vi "pattern_matching_mit_thresholding.vi"() -> ()   [LabVIEW 2014]
uses:
  <vilib>/vision/driver/NI_Vision_Acquisition_Software.lvlib
  <vilib>/userdefined/High Color/IMAQdx.ctl
  <vilib>/vision/NI_Vision_Development_Module.lvlib
  <vilib>/vision/Avi1.llb/AviRefnum.ctl
  <resource>/objmgr/imaqdx.rc
  subvis/Control 1.ctl
panel:
  in  "Replace Value":sgl=1.0 format="%.2f"
  in  "Keep/Replace Value (Replace)":bool=TRUE
  in  "Range":cluster{"Lower value":sgl, "Upper value":sgl}={"Lower value"=128.0, "Upper value"=255.0} {"Upper value" format="%.2f"; "Lower value" format="%.2f"}
  in  "Länge der Spur":i32=50
  in  "Frames Per Second":u32=20
  in  "BayerPattern":u32(ring)=5 items=["None", "GB", "GR", "BG", "RG", "Use Hardware Value"]
  in  "ValueString 2":T1="BayerGB8"
  out "ValueString":string
  out "ValueBool":bool
  out "IPAddress":string
  in  "y":i32
  in  "x":i32
  in  "Pattern2 Farbe":u32(colorbox)=16711680
  in  "pattern3":bool
  in  "y 3":i32
  in  "x 3":i32
  out "Pattern 5":T2(plugin-control)
  in  "Pattern5 Farbe":u32(colorbox)=16711680
  in  "pattern5":bool
  in  "y 5":i32
  in  "x 5":i32
  in  "Pattern4 Farbe":u32(colorbox)=16711680
  in  "pattern4":bool
  in  "y 4":i32
  in  "x 4":i32
  out "Pattern 4":T2(plugin-control)
  in  "Template File Path (Pattern Matching 4":path=path "C:/Users/Kroll/Desktop/Test_04012016/Pattern/templet_invertiert_2.png"
  in  "Template File Path (Pattern Matching 5":path=path "C:/Users/Kroll/Desktop/Test_04012016/Pattern/TEST_PAINT.png"
  in  "Pattern2 Farbe":u32(colorbox)=16711680
  in  "pattern2":bool
  out "Pattern 3":T2(plugin-control)
  in  "Template File Path (Pattern Matching 3":path=path "C:/Users/Kroll/Desktop/Test_04012016/Pattern/pattern3.png"
  out "Pattern1":T2(plugin-control)
  out "Pattern 2":T2(plugin-control)
  in  "Pattern1 Farbe":u32(colorbox)=16711680
  in  "pattern1":bool
  out "Acquired Frames/s":dbl
  in  "Länge des Pfeils":sgl=80.0
  in  "Aufnahme Starten":bool
  out "Selected Path":path
  in  "Max Data Size":u32=10000
  in  "y 2":i32
  in  "x 2":i32
  out "Processed Frames/s":dbl
  in  "Template File Path (Pattern Matching 2":path=path "C:/Users/Kroll/Desktop/Test_04012016/Pattern/pattern_test_1412.png"
  in  "millisecond multiple":u32
  in  "Mittelpunktgröße":sgl
  out "date/time string":string
  in  "file path (dialog if empty)":path=path "I:/123.txt"
  in  "Template File Path (Pattern Matching 1)":path=path "C:/Users/Kroll/Desktop/Test_04012016/Pattern/pattern_1412.png"
  in  "Parameters Pattern":T3={"Number of Matches Requested"=1, "Minimum Match Score"=800.0, "Angle Ranges"=[{"Start Angle"=-180.0, "End Angle"=180.0}, {"Start Angle"=0.0, "End Angle"=360.0}]}
  in  "Programm anhalten":bool
  out "Threshold Image 2":T2(plugin-control)
  out "Image 2":T2(plugin-control)
  # "Speicherort der Log Datei"
  # "Program Delay einstellen"
  # "Zum Rauszoomen Shift benutzen ->"
  # "Aufnahme"
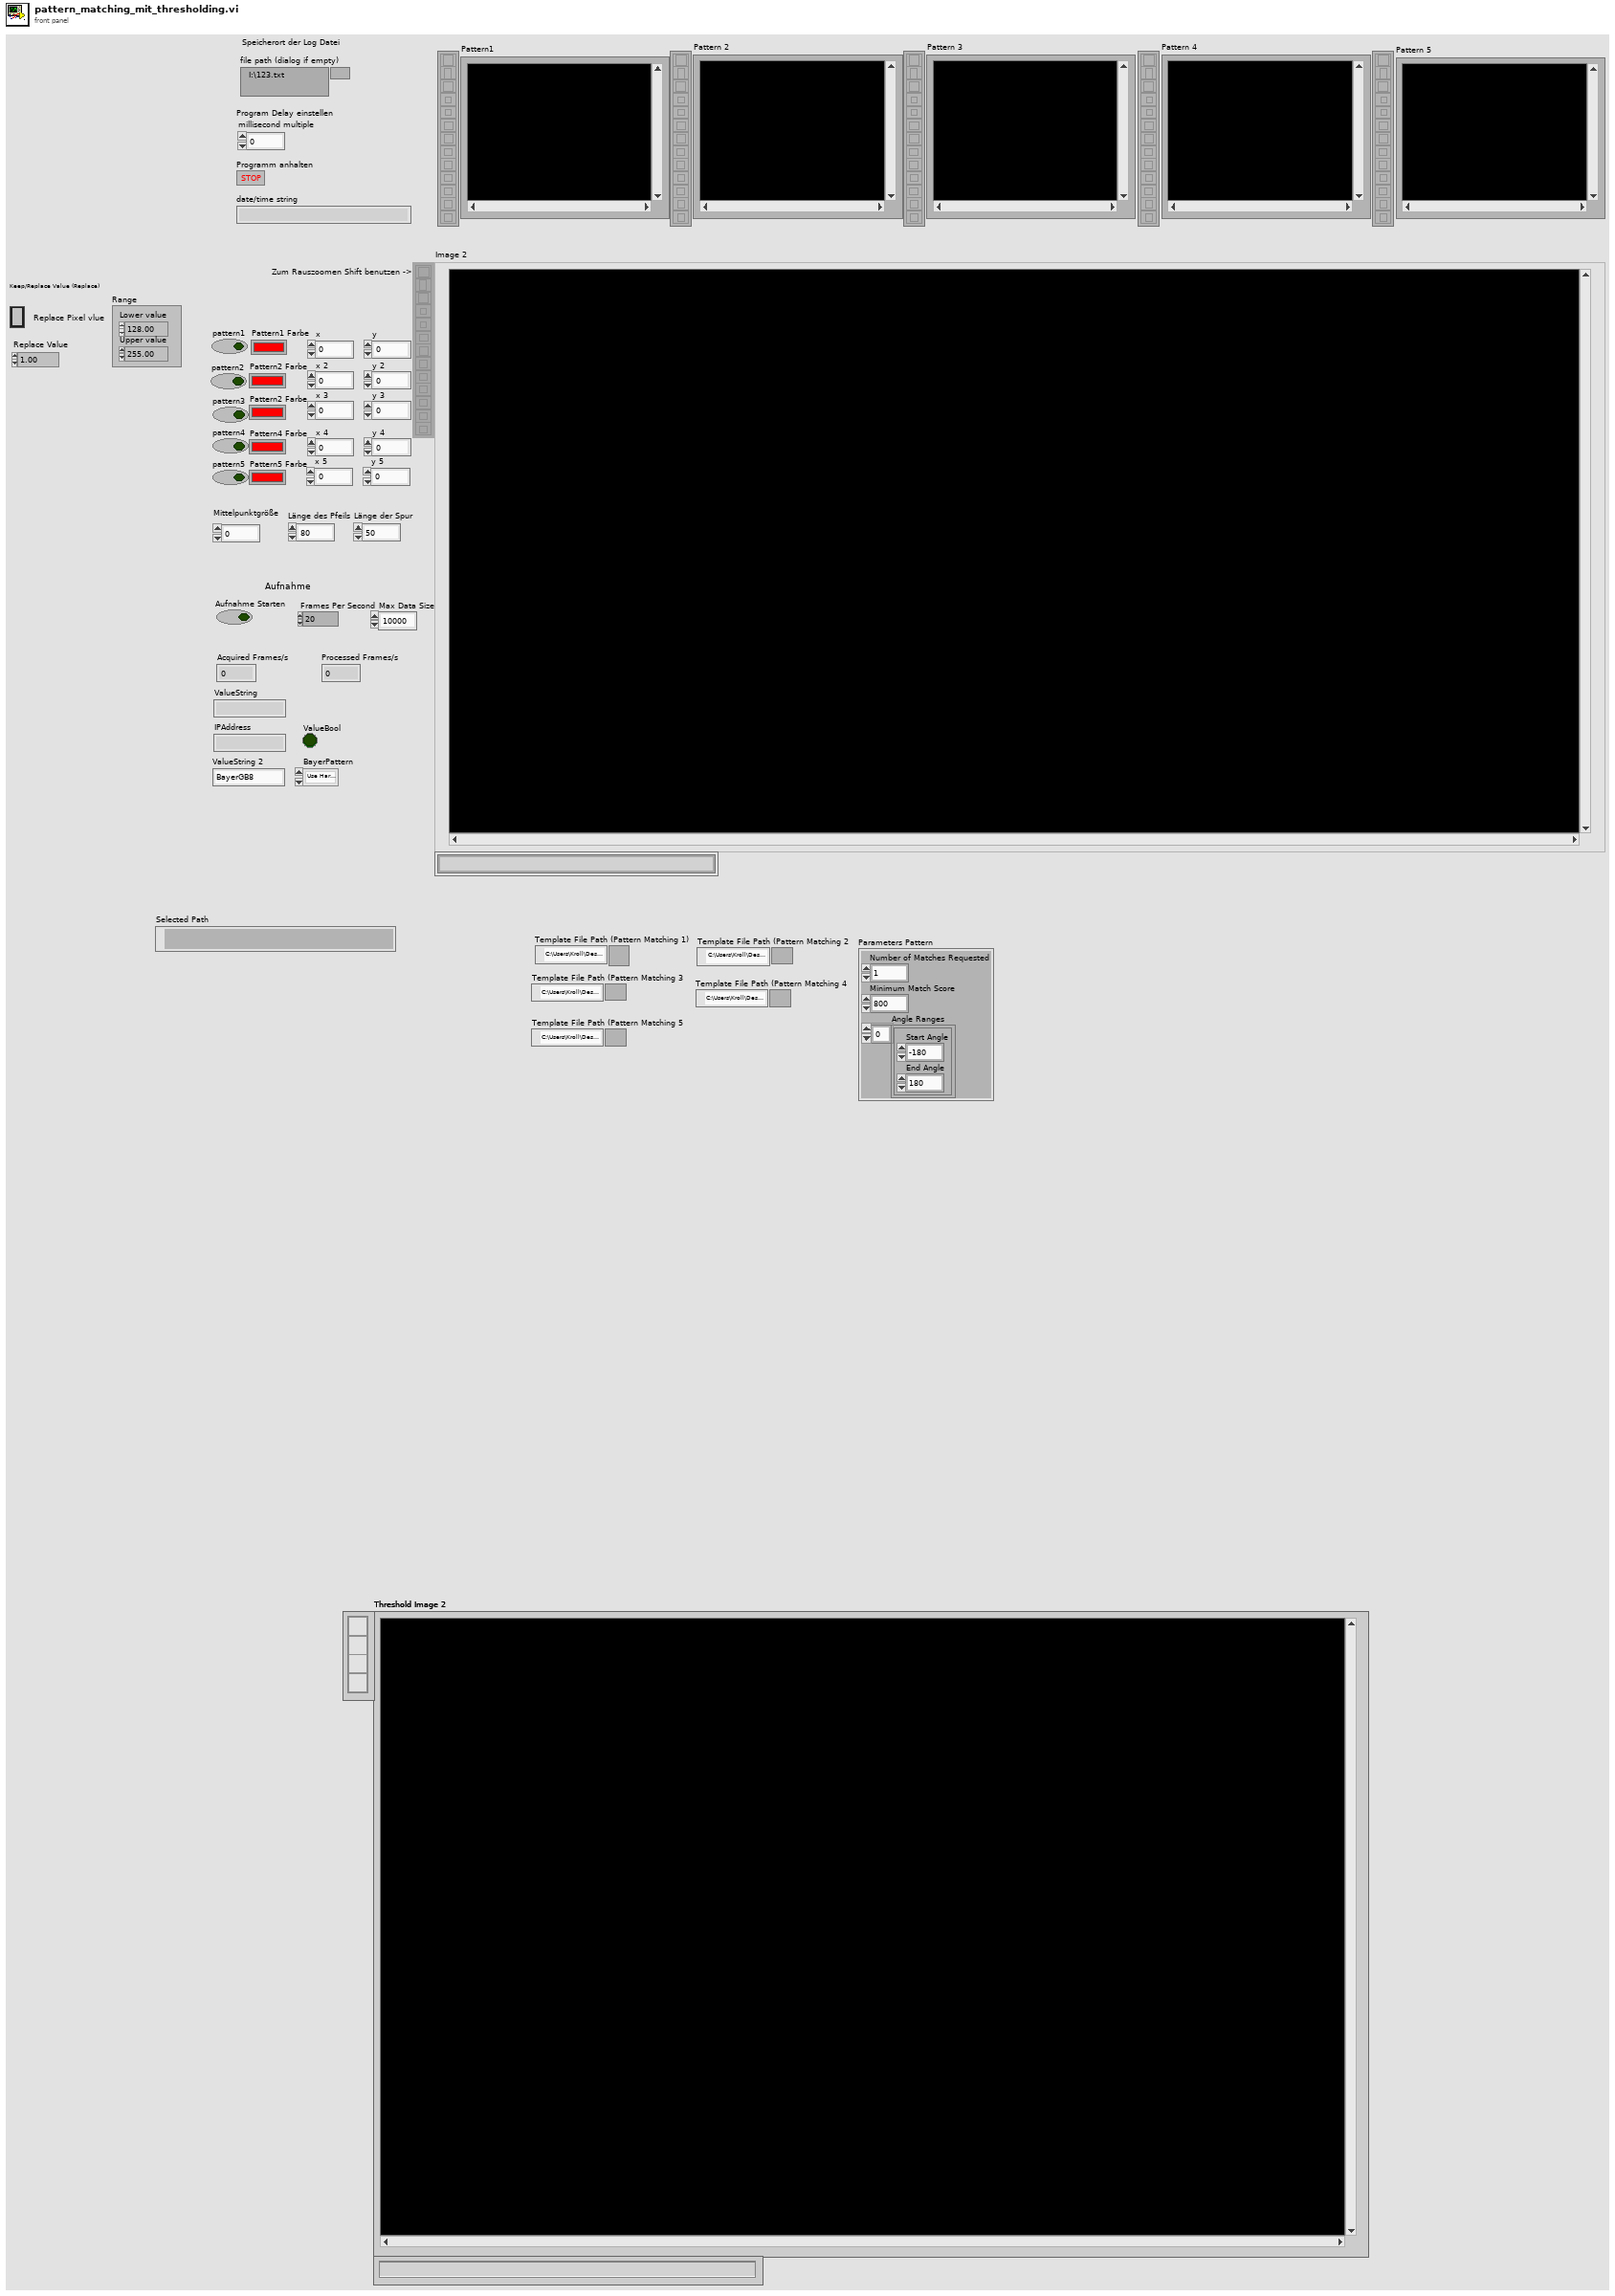
[diagram p1: front panel]
types:
  T1 = typedef "Control 1.ctl" = string
  T2 = typedef "IMAQ Image.ctl" = refnum<image>
  T3 = cluster{"Number of Matches Requested":i32, "Minimum Match Score":sgl, "Angle Ranges":cluster{"Start Angle":sgl, "End Angle":sgl}[]}
  T4 = typedef "IMAQdx.ctl" = refnum<k21>
  T5 = typedef "Image Type" = u32
  T6 = enum16{"open", "replace", "create", "open or create", "replace or create", "replace or create with confirmation"}
  T7 = typedef "AviRefnum.ctl" = refnum<k1>
  T8 = enum32{"existing file", "new file", "new or existing file", "existing dir", "new dir", "new or existing dir", "existing file (use LLBs)", "new file (use LLBs)", "new or existing file (use LLBs)", "new or existing file or directory (use LLBs)"}
  T9 = cluster{"Position":cluster{"x":sgl, "y":sgl}, "Angle":sgl, "Scale":sgl, "Score":sgl, "Bounding Box":cluster{"x":sgl, "y":sgl}[]}[]
  T10 = typedef "ROI Descriptor" = cluster{"Global Rectangle":i32[], "Contours":cluster{"ID":enum32{"External", "Internal"}, "Type":u32, "Coordinates":i32[]}[]}
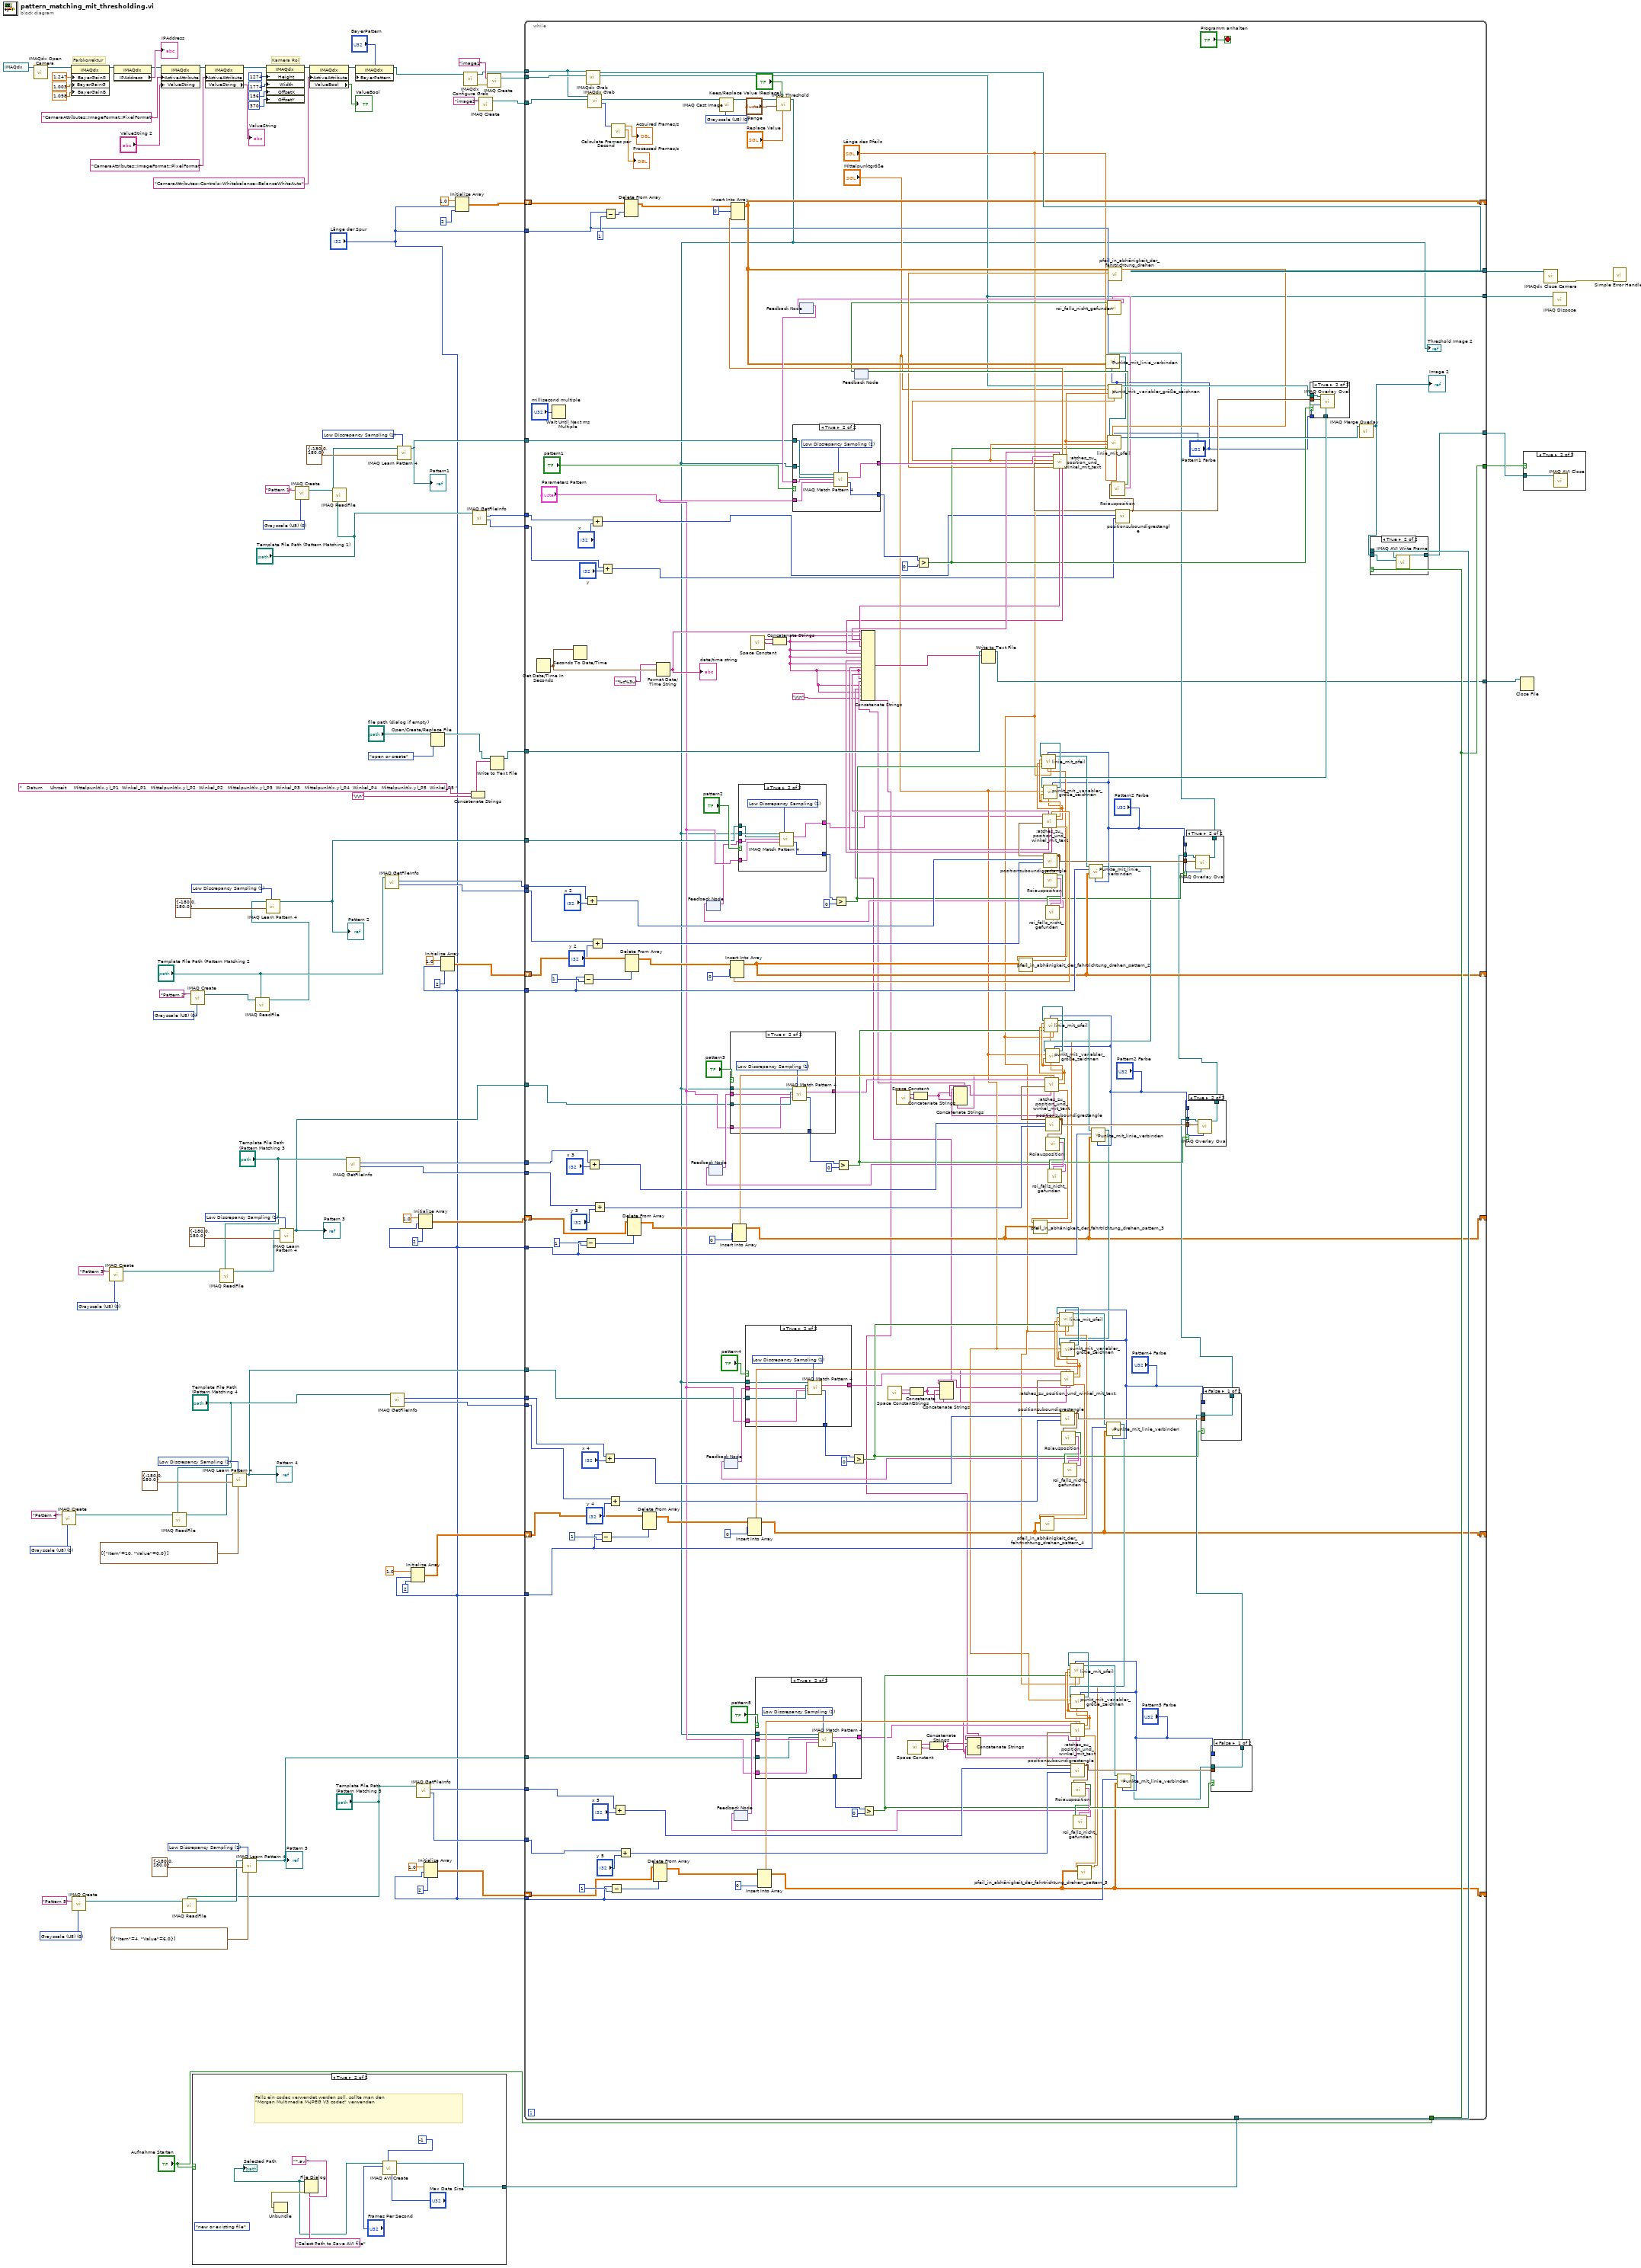
[diagram p0: block diagram]
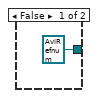
[diagram p3: hidden frame]
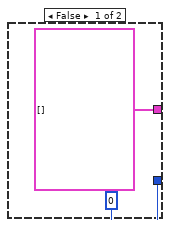
[diagram p4: hidden frame]
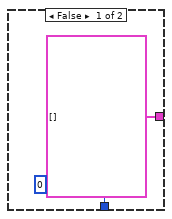
[diagram p5: hidden frame]
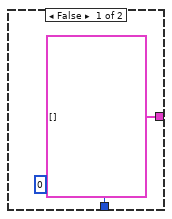
[diagram p7: hidden frame]
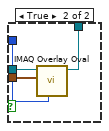
[diagram p8: hidden frame]
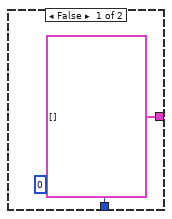
[diagram p9: hidden frame]
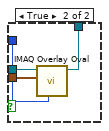
[diagram p10: hidden frame]
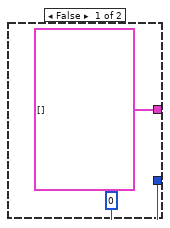
[diagram p11: hidden frame]
diagram:
  w5 = 1 items=["All", "Low Discrepancy Sampling", "Grayscale Value Pyramid", "Gradients Pyramid"] ("Algorithm")
  w35 = T5 0 items=["Grayscale (U8)", "Grayscale (I16)", "Grayscale (SGL)", "Complex (CSG)", "RGB (U32)", "HSL (U32)", "RGB (U64)", "Grayscale (U16)"] ("Image Type")
  w39 = 1 items=["All", "Low Discrepancy Sampling", "Grayscale Value Pyramid", "Gradients Pyramid"] ("Algorithm")
  w44 = T5 0 items=["Grayscale (U8)", "Grayscale (I16)", "Grayscale (SGL)", "Complex (CSG)", "RGB (U32)", "HSL (U32)", "RGB (U64)", "Grayscale (U16)"] ("Image Type")
  w48 = 1 items=["All", "Low Discrepancy Sampling", "Grayscale Value Pyramid", "Gradients Pyramid"] ("Algorithm")
  w62 = T5 0 items=["Grayscale (U8)", "Grayscale (I16)", "Grayscale (SGL)", "Complex (CSG)", "RGB (U32)", "HSL (U32)", "RGB (U64)", "Grayscale (U16)"] ("Image Type")
  w66 = 1 items=["All", "Low Discrepancy Sampling", "Grayscale Value Pyramid", "Gradients Pyramid"] ("Algorithm")
  w75 = T5 0 items=["Grayscale (U8)", "Grayscale (I16)", "Grayscale (SGL)", "Complex (CSG)", "RGB (U32)", "HSL (U32)", "RGB (U64)", "Grayscale (U16)"] ("Image Type")
  w79 = 1 items=["All", "Low Discrepancy Sampling", "Grayscale Value Pyramid", "Gradients Pyramid"] ("Algorithm")
  w81 = T5 0 items=["Grayscale (U8)", "Grayscale (I16)", "Grayscale (SGL)", "Complex (CSG)", "RGB (U32)", "HSL (U32)", "RGB (U64)", "Grayscale (U16)"] ("Image Type")
  # "Kamera Roi"
  # "Farbkorrektur"
  n1 = call <vilib>:"IMAQdx Open Camera.vi"("Session In"=T4 "cam0") -> ("Session Out"=w14:T4)  [unwired: 9 in, 1 out]
  n2 = call "IMAQ Create"("Image Name"="Pattern 4", "Image Type"=w44) -> ("New Image"=w45:T2)  [unwired: 3 in, 1 out]
  n3 = property class="IMAQdx"(reference=w14, "BayerGainR"=1.247, "BayerGainG"=1.003, "BayerGainB"=1.098) -> (reference out=w18:T4)  [unwired: 1 in, 1 out]
  n4 = call "IMAQ Create"("Image Name"="Pattern 5", "Image Type"=w35) -> ("New Image"=w36:T2)  [unwired: 3 in, 1 out]
  n5 = call "IMAQ Create"("Image Name"="Pattern 3", "Image Type"=w62) -> ("New Image"=w63:T2)  [unwired: 3 in, 1 out]
  n6 = property class="IMAQdx"(reference=w18) -> (reference out=w21:T4, "IPAddress"=→"IPAddress":string)  [unwired: 1 in, 1 out]
  n7 = property class="IMAQdx"(reference=w21, "ActiveAttribute"="CameraAttributes::ImageFormat::PixelFormat", "ValueString"="ValueString 2") -> (reference out=w20:T4)  [unwired: 1 in, 1 out]
  n8 = call "IMAQ ReadFile"("File Path"="Template File Path (Pattern Matching 4", "Image"=w45) -> ("Image Out"=w43:T2)  [unwired: 5 in, 4 out]
  n9 = call "IMAQ ReadFile"("File Path"="Template File Path (Pattern Matching 5", "Image"=w36) -> ("Image Out"=w34:T2)  [unwired: 5 in, 4 out]
  n10 = call "IMAQ Create"("Image Name"="Pattern 2", "Image Type"=w81) -> ("New Image"=w82:T2)  [unwired: 3 in, 1 out]
  n11 = case shown="True" "Aufnahme Starten" {
    tunnel: [T7 refnum ("Avi Refnum") w116] -> w87
    frame False {
    }
    frame True {
      (unwired) T8."new or existing file" ("select mode (2)")
      # "Falls ein codec verwendet werden soll, sollte man den \n\"Morgan Multimedia M-JPEG V3 codec\" verwenden"
      n12 = File Dialog(6:"*.avi" ("pattern"), 7:"Select Path to Save AVI file" ("prompt")) -> (0:w119:errorcluster, 3:w118:path)  [unwired: 1 in, 6 out]
      "Selected Path" <- w118
      n13 = Unbundle(w119) -> ()  [unwired: 3 out]
      n14 = call "IMAQ AVI Create"("Max Data Size"="Max Data Size", "quality"=-1, "Frames Per Second"="Frames Per Second", "AVI Path"=w118) -> ("Avi Refnum"=w116:T7)  [unwired: 6 in, 1 out]
    }
  }
  n15 = property class="IMAQdx"(reference=w20, "ActiveAttribute"="CameraAttributes::ImageFormat::PixelFormat") -> (reference out=w10:T4, "ValueString"=→"ValueString":string)  [unwired: 1 in, 1 out]
  n16 = call "IMAQ ReadFile"("File Path"="Template File Path (Pattern Matching 3", "Image"=w63) -> ("Image Out"=w61:T2)  [unwired: 5 in, 4 out]
  n17 = call "IMAQ Learn Pattern 4"("Advanced Options"=cluster{"Item":u16, "Value":dbl}[] [{"Item"=10, "Value"=0.0}], "Algorithm"=w48, "Angle Range"=cluster{"Start Angle":sgl, "End Angle":sgl} {"Start Angle"=-180.0, "End Angle"=180.0}, "Image"=w43) -> ("Template Image Out"=w40:T2)  [unwired: 5 in, 2 out]
  "Pattern 4" <- w40
  n18 = call "IMAQ Learn Pattern 4"("Advanced Options"=cluster{"Item":u16, "Value":dbl}[] [{"Item"=4, "Value"=6.0}], "Algorithm"=w39, "Angle Range"=cluster{"Start Angle":sgl, "End Angle":sgl} {"Start Angle"=-180.0, "End Angle"=180.0}, "Image"=w34) -> ("Template Image Out"=w31:T2)  [unwired: 5 in, 2 out]
  "Pattern 5" <- w31
  n19 = call "IMAQ ReadFile"("File Path"="Template File Path (Pattern Matching 2", "Image"=w82) -> ("Image Out"=w3:T2)  [unwired: 5 in, 4 out]
  n20 = call "IMAQ Learn Pattern 4"("Algorithm"=w5, "Angle Range"=cluster{"Start Angle":sgl, "End Angle":sgl} {"Start Angle"=-180.0, "End Angle"=180.0}, "Image"=w3) -> ("Template Image Out"=w2:T2)  [unwired: 6 in, 2 out]
  "Pattern 2" <- w2
  n21 = property class="IMAQdx"(reference=w10, "Height"=u32 1274, "Width"=u32 1774, "OffsetX"=u32 156, "OffsetY"=u32 370) -> (reference out=w11:T4)  [unwired: 1 in, 1 out]
  n22 = call "IMAQ Learn Pattern 4"("Algorithm"=w66, "Angle Range"=cluster{"Start Angle":sgl, "End Angle":sgl} {"Start Angle"=-180.0, "End Angle"=180.0}, "Image"=w61) -> ("Template Image Out"=w59:T2)  [unwired: 6 in, 2 out]
  "Pattern 3" <- w59
  n23 = call "IMAQ Create"("Image Name"="Pattern 1", "Image Type"=w75) -> ("New Image"=w76:T2)  [unwired: 3 in, 1 out]
  n24 = property class="IMAQdx"(reference=w11, "ActiveAttribute"="CameraAttributes::Controls::Whitebalance::BalanceWhiteAuto") -> (reference out=w26:T4, "ValueBool"=→"ValueBool":bool)  [unwired: 1 in, 1 out]
  n25 = call "IMAQ ReadFile"("File Path"="Template File Path (Pattern Matching 1)", "Image"=w76) -> ("Image Out"=w73:T2)  [unwired: 5 in, 4 out]
  n26 = call "IMAQ GetFileInfo"("File Path"="Template File Path (Pattern Matching 3") -> ("Y Resolution"=w67:i32, "X Resolution"=w68:i32)  [unwired: 4 in, 5 out]
  n27 = property class="IMAQdx"(reference=w26, "BayerPattern"="BayerPattern") -> (reference out=w12:T4)  [unwired: 1 in, 1 out]
  n28 = call "IMAQ GetFileInfo"("File Path"="Template File Path (Pattern Matching 2") -> ("Y Resolution"=w92:i32, "X Resolution"=w93:i32)  [unwired: 4 in, 5 out]
  n29 = call "IMAQ GetFileInfo"("File Path"="Template File Path (Pattern Matching 4") -> ("Y Resolution"=w54:i32, "X Resolution"=w55:i32)  [unwired: 4 in, 5 out]
  n30 = call "IMAQ Learn Pattern 4"("Algorithm"=w79, "Angle Range"=cluster{"Start Angle":sgl, "End Angle":sgl} {"Start Angle"=-180.0, "End Angle"=180.0}, "Image"=w73) -> ("Template Image Out"=w72:T2)  [unwired: 6 in, 2 out]
  "Pattern1" <- w72
  n31 = Initialize Array "Initialize Array"(1.0 ("element"), "Länge der Spur", 2 ("dimension size")) -> (w56:dbl[][])
  n32 = call "IMAQ GetFileInfo"("File Path"="Template File Path (Pattern Matching 5") -> ("Y Resolution"=w49:i32, "X Resolution"=w50:i32)  [unwired: 4 in, 5 out]
  n33 = Initialize Array "Initialize Array"(1.0 ("element"), "Länge der Spur", 2 ("dimension size")) -> (w69:dbl[][])
  n34 = Initialize Array "Initialize Array"(1.0 ("element"), "Länge der Spur", 2 ("dimension size")) -> (w51:dbl[][])
  n35 = Open/Create/Replace File(file path (use dialog)="file path (dialog if empty)", operation (0:open)=T6."open or create") -> (refnum out=w100:refnum<file>)  [unwired: 4 in, 2 out]
  n36 = Initialize Array "Initialize Array"(1.0 ("element"), "Länge der Spur", 2 ("dimension size")) -> (w89:dbl[][])
  n37 = Initialize Array "Initialize Array"(1.0 ("element"), "Länge der Spur", 2 ("dimension size")) -> (w95:dbl[][])
  n38 = call <vilib>:"IMAQdx Configure Grab.vi"("Session In"=w12) -> ("error out"=w113:errorcluster, "Session Out"=w111:T4)  [unwired: 9 in]
  n39 = Concatenate Strings("   Datum     Uhrzeit     Mittelpunkt(x,y)_P1  Winkel_P1   Mittelpunkt(x,y)_P2  Winkel_P2   Mittelpunkt(x,y)_P3  Winkel_P3   Mittelpunkt(x,y)_P4  Winkel_P4   Mittelpunkt(x,y)_P5  Winkel_P5 " ("string"), "\r\n") -> (w97:string)
  n40 = call "IMAQ GetFileInfo"("File Path"="Template File Path (Pattern Matching 1)") -> ("Y Resolution"=w103:i32, "X Resolution"=w104:i32)  [unwired: 4 in, 5 out]
  n41 = call "IMAQ Create"("Image Name"="image2") -> ("New Image"=w106:T2)  [unwired: 4 in, 1 out]
  n42 = call "IMAQ Create"("Image Name"="image1", "error in (no error)"=w113) -> ("New Image"=w110:T2)  [unwired: 3 in, 1 out]
  n43 = Write to Text File(file (use dialog)=w100, text=w97) -> (refnum out=w99:refnum<file>)  [unwired: 2 in, 2 out]
  n44 = while {
    tunnel: w111 -> [w353]
    tunnel: w110 -> [w354]
    tunnel: [w355] -> w108
    tunnel: [w128] -> w105
    tunnel: w106 -> [w352]
    tunnel: w104 -> [w159]
    tunnel: w103 -> [w161]
    tunnel: w99 -> [w348]
    shift-right: [w286] -> _
    shift-left: w95 -> [w339]
    tunnel: "Länge der Spur" -> [w328]
    tunnel: w93 -> [w325]
    tunnel: w92 -> [w323]
    tunnel: "Länge der Spur" -> [w318]
    shift-right: [w291] -> _
    shift-left: w89 -> [w330]
    tunnel: w87 -> [w311]
    tunnel: [w310] -> w86
    tunnel: "Aufnahme Starten" -> [w302]
    tunnel: [w302] -> w84
    tunnel: w2 -> [w133]
    tunnel: w72 -> [w275]
    tunnel: "Länge der Spur" -> [w173]
    shift-right: [w165] -> _
    shift-left: w69 -> [w174]
    tunnel: w68 -> [w176]
    tunnel: w67 -> [w175]
    tunnel: w59 -> [w177]
    tunnel: "Länge der Spur" -> [w241]
    tunnel: w55 -> [w245]
    tunnel: w54 -> [w243]
    shift-right: [w204] -> _
    shift-left: w56 -> [w242]
    tunnel: "Länge der Spur" -> [w213]
    shift-right: [w208] -> _
    shift-left: w51 -> [w214]
    tunnel: w50 -> [w216]
    tunnel: w49 -> [w215]
    tunnel: w40 -> [w244]
    tunnel: w31 -> [w136]
    tunnel: [w209] -> w30
    stop <- "Programm anhalten" stop-if-true
    w281 = T5 0 items=["Grayscale (U8)", "Grayscale (I16)", "Grayscale (SGL)", "Complex (CSG)", "RGB (U32)", "HSL (U32)", "RGB (U64)", "Grayscale (U16)"] ("Image Type")
    n45 = Get Date/Time In Seconds() -> (seconds since 1Jan1904=w347:timestamp)
    n46 = Wait Until Next ms Multiple(millisecond multiple="millisecond multiple") -> ()  [unwired: 1 out]
    n47 = Seconds To Date/Time(time stamp (now)=w347) -> ()  [unwired: 1 in, 1 out]
    n48 = Subtract(x=w318, y=1) -> (x-y=w331:i32)
    n49 = Subtract(x=w173, y=1) -> (x-y=w199:i32)
    n50 = Add(x=w325, y="x 2") -> (x+y=w326:i32)
    n51 = call <vilib>:"IMAQdx Grab.vi"("Image In"=w354, "Session In"=w353) -> ("Image Out"=w128:T2, "Session Out"=w355:T4)  [unwired: 6 in, 2 out]
    n52 = Add(x=w176, y="x 3") -> (x+y=w198:i32)
    n53 = call <vilib>:"IMAQdx Grab.vi"("Image In"=w352, "Session In"=w353) -> ("Buffer Number Out"=w350:u32, "Image Out"=w129:T2)  [unwired: 6 in, 2 out]
    n54 = Add(x=w159, y="x") -> (x+y=w158:i32)
    n55 = Add(x=w323, y="y 2") -> (x+y=w321:i32)
    n56 = Add(x=w175, y="y 3") -> (x+y=w195:i32)
    n57 = Subtract(x=w241, y=1) -> (x-y=w267:i32)
    n58 = Add(x=w161, y="y") -> (x+y=w160:i32)
    n59 = Add(x=w245, y="x 4") -> (x+y=w266:i32)
    n60 = Subtract(x=w328, y=1) -> (x-y=w335:i32)
    n61 = Add(x=w243, y="y 4") -> (x+y=w263:i32)
    n62 = Subtract(x=w213, y=1) -> (x-y=w237:i32)
    n63 = call <vilib>:"Calculate Frames per Second.vi"("Buffer Number"=w350) -> ("Processed Frames/s"=→"Processed Frames/s":dbl, "Acquired Frames/s"=→"Acquired Frames/s":dbl)  [unwired: 8 in, 1 out]
    n64 = Add(x=w216, y="x 5") -> (x+y=w236:i32)
    n65 = Add(x=w215, y="y 5") -> (x+y=w233:i32)
    n66 = Delete From Array "Delete From Array"(array=w339, index (row)=w335) -> (array with subset deleted=w338:dbl[][])  [unwired: 2 in, 1 out]
    n67 = Delete From Array "Delete From Array"(array=w330, index (row)=w331) -> (array with subset deleted=w334:dbl[][])  [unwired: 2 in, 1 out]
    n68 = Delete From Array "Delete From Array"(array=w174, index (row)=w199) -> (array with subset deleted=w202:dbl[][])  [unwired: 2 in, 1 out]
    n69 = Delete From Array "Delete From Array"(array=w242, index (row)=w267) -> (array with subset deleted=w270:dbl[][])  [unwired: 2 in, 1 out]
    n70 = Delete From Array "Delete From Array"(array=w214, index (row)=w237) -> (array with subset deleted=w240:dbl[][])  [unwired: 2 in, 1 out]
    n71 = Format Date/Time String(time format string (%c)="%c%3u", seconds (now)=w347) -> (date/time string=w345:string)  [unwired: 1 in]
    "date/time string" <- w345
    n72 = feedback #1() -> (w131:T10)  [unwired: 1 in]
    n73 = feedback #2() -> (w183:T10)  [unwired: 1 in]
    n74 = call "IMAQ Cast Image"("Image Type"=w281, "Image Src"=w129) -> ("Image Dst Out"=w127:T2)  [unwired: 8 in, 1 out]
    n75 = feedback #3() -> (w251:T10)  [unwired: 1 in]
    n76 = feedback #4() -> (w137:T10)  [unwired: 1 in]
    n77 = call <vilib>:"Space Constant.vi"() -> ("String"=w272:string)
    n78 = Concatenate Strings(w272, w272) -> (w140:string)
    n79 = call "IMAQ Threshold"("Replace Value"="Replace Value", "Keep/Replace Value (Replace)"="Keep/Replace Value (Replace)", "Range"="Range", "Image Src"=w127) -> ("Image Dst Out"=w126:T2)  [unwired: 6 in, 1 out]
    "Threshold Image 2" <- w126
    n80 = case shown="True" "pattern3" {
      tunnel: w177 -> [_ w373]
      tunnel: w183 -> [_ w371]
      tunnel: "Parameters Pattern" -> [_ w370]
      tunnel: [0 ("Number of Matches") w369] -> w182
      tunnel: [T9 [] ("Matches (pixel)") w368] -> w181
      tunnel: w126 -> [_ w367]
      frame False {
      }
      frame True {
        w372 = 1 items=["All", "Low Discrepancy Sampling", "Grayscale Value Pyramid", "Gradients Pyramid"] ("Algorithm")
        n81 = call "IMAQ Match Pattern 4"("Image"=w367, "Algorithm"=w372, "Template Image"=w373, "ROI Descriptor"=w371, "Parameters"=w370) -> ("Matches (pixel)"=w368:T9, "Number of Matches"=w369:i32)  [unwired: 6 in, 3 out]
      }
    }
    n82 = case shown="True" "pattern2" {
      tunnel: [0 ("Number of Matches (Pattern Matching 1)") w361] -> w130
      tunnel: w133 -> [_ w358]
      tunnel: w131 -> [_ w364]
      tunnel: [T9 [] ("Matches (Pattern Matching 1)") w362] -> w135
      tunnel: "Parameters Pattern" -> [_ w363]
      tunnel: w126 -> [_ w359]
      frame False {
      }
      frame True {
        w360 = 1 items=["All", "Low Discrepancy Sampling", "Grayscale Value Pyramid", "Gradients Pyramid"] ("Algorithm")
        n83 = call "IMAQ Match Pattern 4"("Image"=w359, "Algorithm"=w360, "Template Image"=w358, "ROI Descriptor"=w364, "Parameters"=w363) -> ("Matches (pixel)"=w362:T9, "Number of Matches"=w361:i32)  [unwired: 6 in, 3 out]
      }
    }
    n84 = case shown="True" "pattern4" {
      tunnel: w244 -> [_ w401]
      tunnel: w251 -> [_ w399]
      tunnel: "Parameters Pattern" -> [_ w398]
      tunnel: [0 ("Number of Matches") w397] -> w250
      tunnel: [T9 [] ("Matches (pixel)") w396] -> w249
      tunnel: w126 -> [_ w395]
      frame False {
      }
      frame True {
        w400 = 1 items=["All", "Low Discrepancy Sampling", "Grayscale Value Pyramid", "Gradients Pyramid"] ("Algorithm")
        n85 = call "IMAQ Match Pattern 4"("Image"=w395, "Algorithm"=w400, "Template Image"=w401, "ROI Descriptor"=w399, "Parameters"=w398) -> ("Matches (pixel)"=w396:T9, "Number of Matches"=w397:i32)  [unwired: 6 in, 3 out]
      }
    }
    n86 = case shown="True" "pattern5" {
      tunnel: w137 -> [_ w386]
      tunnel: "Parameters Pattern" -> [_ w385]
      tunnel: [0 ("Number of Matches") w384] -> w221
      tunnel: [T9 [] ("Matches (pixel)") w383] -> w220
      tunnel: w136 -> [_ w382]
      tunnel: w126 -> [_ w381]
      frame False {
      }
      frame True {
        w387 = 1 items=["All", "Low Discrepancy Sampling", "Grayscale Value Pyramid", "Gradients Pyramid"] ("Algorithm")
        n87 = call "IMAQ Match Pattern 4"("Image"=w381, "Algorithm"=w387, "Template Image"=w382, "ROI Descriptor"=w386, "Parameters"=w385) -> ("Matches (pixel)"=w383:T9, "Number of Matches"=w384:i32)  [unwired: 6 in, 3 out]
      }
    }
    n88 = feedback #5() -> (w307:T10)  [unwired: 1 in]
    n89 = case shown="True" "pattern1" {
      tunnel: [0 ("Number of Matches (Pattern Matching 1)") w410] -> w284
      tunnel: w126 -> [_ w415]
      tunnel: w307 -> [_ w413]
      tunnel: [T9 [] ("Matches (Pattern Matching 1)") w411] -> w300
      tunnel: "Parameters Pattern" -> [_ w412]
      tunnel: w275 -> [_ w414]
      frame False {
      }
      frame True {
        w409 = 1 items=["All", "Low Discrepancy Sampling", "Grayscale Value Pyramid", "Gradients Pyramid"] ("Algorithm")
        n90 = call "IMAQ Match Pattern 4"("Image"=w415, "Algorithm"=w409, "Template Image"=w414, "ROI Descriptor"=w413, "Parameters"=w412) -> ("Matches (pixel)"=w411:T9, "Number of Matches"=w410:i32)  [unwired: 6 in, 3 out]
      }
    }
    n91 = Greater?(x=w130, y=0) -> (0:w282:bool)
    n92 = Greater?(x=w182, y=0) -> (0:w184:bool)
    n93 = Greater?(x=w250, y=0) -> (0:w252:bool)
    n94 = feedback #6() -> (w278:bool)  [unwired: 1 in]
    n95 = Greater?(x=w221, y=0) -> (0:w222:bool)
    n96 = call <vilib>:"Space Constant.vi"() -> ("String"=w153:string)
    n97 = call <vilib>:"Space Constant.vi"() -> ("String"=w154:string)
    n98 = call <vilib>:"Space Constant.vi"() -> ("String"=w148:string)
    n99 = Concatenate Strings(w153, w153) -> (w149:string)
    n100 = Concatenate Strings(w154, w154) -> (w143:string)
    n101 = Greater?(x=w284, y=0) -> (0:w283:bool)
    n102 = Concatenate Strings(w148, w148) -> (w144:string)
    n103 = call ";atches_zu_position_und_winkel_mit_text.vi"("Matches (Pattern Matching 1)"=w135) -> ("Angle"=w288:sgl, "Position"=w316:cluster{"x":sgl, "y":sgl}, "x"=w296:sgl, "y"=w297:sgl, "String"=w313:string, "Array"=w317:sgl[], "String 2"=w314:string, "String 3"=w315:string)  [unwired: 3 in]
    n104 = Insert Into Array "Insert Into Array"(array=w334, index (row)=0 ("index"), new element=w317) -> (w291:dbl[][])  [unwired: 1 in]
    n105 = call "pfeil_in_abhänigkeit_der_fahrtrichtung_drehen_pattern_2.vi"("Array"=w291, "Angle in"=w288) -> ("Angle out"=w287:sgl)  [unwired: 9 in]
    n106 = call "positionzuboundigrectangle.vi"("Y Resolution"=w321, "X Resolution"=w326, "Position"=w316) -> ("Cluster"=w306:cluster{dbl, dbl, dbl, dbl})  [unwired: 8 in]
    n107 = call "Roiausposition.vi"("Cluster"=w306) -> ("ROI Descriptor"=w305:T10, "Boolean"=w304:bool)  [unwired: 9 in]
    n108 = call ";atches_zu_position_und_winkel_mit_text.vi"("Matches (Pattern Matching 1)"=w181) -> ("Angle"=w166:sgl, "Position"=w192:cluster{"x":sgl, "y":sgl}, "x"=w185:sgl, "y"=w186:sgl, "String"=w157:string, "Array"=w193:sgl[], "String 2"=w156:string, "String 3"=w155:string)  [unwired: 3 in]
    n109 = Insert Into Array "Insert Into Array"(array=w202, index (row)=0 ("index"), new element=w193) -> (w165:dbl[][])  [unwired: 1 in]
    n110 = Concatenate Strings(w157, w143, w156, w143, w155) -> (w142:string)
    n111 = call "pfeil_in_abhänigkeit_der_fahrtrichtung_drehen_pattern_3.vi"("Array"=w165, "Angle in"=w166) -> ("Angle out"=w164:sgl)  [unwired: 9 in]
    n112 = call "roi_falls_nicht_gefunden.vi"("ROI Descriptor in"=w305, "Boolean"=w304) -> ("ROI Descriptor out"=w303:T10)  [unwired: 9 in]
    n113 = feedback-in #1(w303) -> ()
    n114 = call "positionzuboundigrectangle.vi"("Y Resolution"=w195, "X Resolution"=w198, "Position"=w192) -> ("Cluster"=w191:cluster{dbl, dbl, dbl, dbl})  [unwired: 8 in]
    n115 = call "Roiausposition.vi"("Cluster"=w191) -> ("ROI Descriptor"=w190:T10, "Boolean"=w189:bool)  [unwired: 9 in]
    n116 = call "roi_falls_nicht_gefunden.vi"("ROI Descriptor in"=w190, "Boolean"=w189) -> ("ROI Descriptor out"=w188:T10)  [unwired: 9 in]
    n117 = feedback-in #2(w188) -> ()
    n118 = call ";atches_zu_position_und_winkel_mit_text.vi"("Matches (Pattern Matching 1)"=w300) -> ("Angle"=w280:sgl, "Position"=w309:cluster{"x":sgl, "y":sgl}, "x"=w293:sgl, "y"=w292:sgl, "String"=w341:string, "Array"=w329:sgl[], "String 2"=w342:string, "String 3"=w343:string)  [unwired: 3 in]
    n119 = Insert Into Array "Insert Into Array"(array=w338, index (row)=0 ("index"), new element=w329) -> (w286:dbl[][])  [unwired: 1 in]
    n120 = call ";atches_zu_position_und_winkel_mit_text.vi"("Matches (Pattern Matching 1)"=w249) -> ("Angle"=w205:sgl, "Position"=w260:cluster{"x":sgl, "y":sgl}, "x"=w253:sgl, "y"=w254:sgl, "String"=w152:string, "Array"=w261:sgl[], "String 2"=w151:string, "String 3"=w150:string)  [unwired: 3 in]
    n121 = Insert Into Array "Insert Into Array"(array=w270, index (row)=0 ("index"), new element=w261) -> (w204:dbl[][])  [unwired: 1 in]
    n122 = Concatenate Strings(w152, w149, w151, w149, w150) -> (w141:string)
    n123 = call "pfeil_in_abhänigkeit_der_fahrtrichtung_drehen_pattern_4.vi"("Array"=w204, "Angle in"=w205) -> ("Angle out"=w203:sgl)  [unwired: 9 in]
    n124 = call "positionzuboundigrectangle.vi"("Y Resolution"=w263, "X Resolution"=w266, "Position"=w260) -> ("Cluster"=w259:cluster{dbl, dbl, dbl, dbl})  [unwired: 8 in]
    n125 = call "Roiausposition.vi"("Cluster"=w259) -> ("ROI Descriptor"=w258:T10, "Boolean"=w257:bool)  [unwired: 9 in]
    n126 = call "roi_falls_nicht_gefunden.vi"("ROI Descriptor in"=w258, "Boolean"=w257) -> ("ROI Descriptor out"=w256:T10)  [unwired: 9 in]
    n127 = feedback-in #3(w256) -> ()
    n128 = call ";atches_zu_position_und_winkel_mit_text.vi"("Matches (Pattern Matching 1)"=w220) -> ("Angle"=w206:sgl, "Position"=w230:cluster{"x":sgl, "y":sgl}, "x"=w223:sgl, "y"=w224:sgl, "String"=w147:string, "Array"=w231:sgl[], "String 2"=w146:string, "String 3"=w145:string)  [unwired: 3 in]
    n129 = Insert Into Array "Insert Into Array"(array=w240, index (row)=0 ("index"), new element=w231) -> (w208:dbl[][])  [unwired: 1 in]
    n130 = Concatenate Strings(w147, w144, w146, w144, w145) -> (w139:string)
    n131 = Concatenate Strings(w345, w140, w343, w140, w342, w140, w341, w140, w313, w140, w314, w140, w315, w140, w142, w140, w141, w140, w139, "\r\n") -> (w344:string)
    n132 = Write to Text File(file (use dialog)=w348, text=w344) -> (refnum out=w209:refnum<file>)  [unwired: 2 in, 2 out]
    n133 = call "positionzuboundigrectangle.vi"("Y Resolution"=w233, "X Resolution"=w236, "Position"=w230) -> ("Cluster"=w229:cluster{dbl, dbl, dbl, dbl})  [unwired: 8 in]
    n134 = call "Roiausposition.vi"("Cluster"=w229) -> ("ROI Descriptor"=w228:T10, "Boolean"=w227:bool)  [unwired: 9 in]
    n135 = call "roi_falls_nicht_gefunden.vi"("ROI Descriptor in"=w228, "Boolean"=w227) -> ("ROI Descriptor out"=w226:T10)  [unwired: 9 in]
    n136 = feedback-in #4(w226) -> ()
    n137 = call "pfeil_in_abhänigkeit_der_fahrtrichtung_drehen_pattern_5.vi"("Array"=w208, "Angle in"=w206) -> ("Angle out"=w207:sgl)  [unwired: 9 in]
    n138 = call "pfeil_in_abhänigkeit_der_fahrtrichtung_drehen.vi"("Angle in"=w280, "Array"=w286) -> ("Angle out"=w285:sgl)  [unwired: 9 in]
    n139 = call "punkt_mit _variabler_größe_zeichnen.vi"("Color"="Pattern1 Farbe", "x"=w293, "y"=w292, "größe"="Mittelpunktgröße", "Refnum in"=w128) -> ("Refnum out"=w327:T2)  [unwired: 5 in, 1 out]
    n140 = call "positionzuboundigrectangle.vi"("Y Resolution"=w160, "X Resolution"=w158, "Position"=w309) -> ("Cluster"=w301:cluster{dbl, dbl, dbl, dbl})  [unwired: 8 in]
    n141 = call "Roiausposition.vi"("Cluster"=w301) -> ("ROI Descriptor"=w276:T10, "Boolean"=w308:bool)  [unwired: 9 in]
    n142 = feedback-in #6(w308) -> ()
    n143 = call "roi_falls_nicht_gefunden.vi"("ROI Descriptor in"=w276, "Boolean"=w278) -> ("ROI Descriptor out"=w277:T10)  [unwired: 9 in]
    n144 = feedback-in #5(w277) -> ()
    n145 = case shown="True" w283 {
      tunnel: w301 -> [_ w429]
      tunnel: [w425 w428] -> w299
      tunnel: w327 -> [w425 w427]
      tunnel: "Pattern1 Farbe" -> [_ w426]
      frame False {
      }
      frame True {
        n146 = call "IMAQ Overlay Oval"("Color"=w426, "Bounding Rectangle"=w429, "Image"=w427) -> ("Image Out"=w428:T2)  [unwired: 7 in, 1 out]
      }
    }
    n147 = call "punkt_mit _variabler_größe_zeichnen.vi"("Color"="Pattern2 Farbe", "x"=w296, "y"=w297, "größe"="Mittelpunktgröße", "Refnum in"=w299) -> ("Refnum out"=w298:T2)  [unwired: 5 in, 1 out]
    n148 = call "linie_mit_pfeil.vi"("Richtungspfeillänge"="Länge des Pfeils", "Angle"=w287, "Color"="Pattern2 Farbe", "Boolean"=w282, "x"=w296, "y"=w297, "Refnum in"=w298) -> ("Refnum out"=w274:T2)  [unwired: 4 in]
    n149 = call "Punkte_mit_linie_verbinden.vi"("Color"="Pattern2 Farbe", "Array"=w291, "dimension size"=w318, "Refnum in"=w274) -> ("Refnum out"=w170:T2)  [unwired: 7 in]
    n150 = call "punkt_mit _variabler_größe_zeichnen.vi"("Color"="Pattern2 Farbe", "x"=w185, "y"=w186, "größe"="Mittelpunktgröße", "Refnum in"=w170) -> ("Refnum out"=w187:T2)  [unwired: 5 in, 1 out]
    n151 = call "linie_mit_pfeil.vi"("Richtungspfeillänge"="Länge des Pfeils", "Angle"=w164, "Color"="Pattern2 Farbe", "Boolean"=w184, "x"=w185, "y"=w186, "Refnum in"=w187) -> ("Refnum out"=w180:T2)  [unwired: 4 in]
    n152 = call "Punkte_mit_linie_verbinden.vi"("Color"="Pattern2 Farbe", "Array"=w165, "dimension size"=w173, "Refnum in"=w180) -> ("Refnum out"=w171:T2)  [unwired: 7 in]
    n153 = call "punkt_mit _variabler_größe_zeichnen.vi"("Color"="Pattern4 Farbe", "x"=w253, "y"=w254, "größe"="Mittelpunktgröße", "Refnum in"=w171) -> ("Refnum out"=w255:T2)  [unwired: 5 in, 1 out]
    n154 = call "linie_mit_pfeil.vi"("Richtungspfeillänge"="Länge des Pfeils", "Angle"=w203, "Color"="Pattern4 Farbe", "Boolean"=w252, "x"=w253, "y"=w254, "Refnum in"=w255) -> ("Refnum out"=w248:T2)  [unwired: 4 in]
    n155 = call "Punkte_mit_linie_verbinden.vi"("Color"="Pattern4 Farbe", "Array"=w204, "dimension size"=w241, "Refnum in"=w248) -> ("Refnum out"=w212:T2)  [unwired: 7 in]
    n156 = call "punkt_mit _variabler_größe_zeichnen.vi"("Color"="Pattern5 Farbe", "x"=w223, "y"=w224, "größe"="Mittelpunktgröße", "Refnum in"=w212) -> ("Refnum out"=w225:T2)  [unwired: 5 in, 1 out]
    n157 = call "linie_mit_pfeil.vi"("Richtungspfeillänge"="Länge des Pfeils", "Angle"=w207, "Color"="Pattern5 Farbe", "Boolean"=w222, "x"=w223, "y"=w224, "Refnum in"=w225) -> ("Refnum out"=w219:T2)  [unwired: 4 in]
    n158 = call "Punkte_mit_linie_verbinden.vi"("Color"="Pattern5 Farbe", "Array"=w208, "dimension size"=w213, "Refnum in"=w219) -> ("Refnum out"=w210:T2)  [unwired: 7 in]
    n159 = case shown="False" w222 {
      tunnel: w229 -> [_ w392]
      tunnel: w210 -> [w388 w391]
      tunnel: [w388 w390] -> w211
      tunnel: "Pattern5 Farbe" -> [_ w389]
      frame False {
      }
      frame True {
        n160 = call "IMAQ Overlay Oval"("Color"=w389, "Bounding Rectangle"=w392, "Image"=w391) -> ("Image Out"=w390:T2)  [unwired: 7 in, 1 out]
      }
    }
    n161 = case shown="False" w252 {
      tunnel: w259 -> [_ w406]
      tunnel: w211 -> [w402 w405]
      tunnel: [w402 w404] -> w169
      tunnel: "Pattern4 Farbe" -> [_ w403]
      frame False {
      }
      frame True {
        n162 = call "IMAQ Overlay Oval"("Color"=w403, "Bounding Rectangle"=w406, "Image"=w405) -> ("Image Out"=w404:T2)  [unwired: 7 in, 1 out]
      }
    }
    n163 = case shown="True" w184 {
      tunnel: w191 -> [_ w378]
      tunnel: [w374 w377] -> w172
      tunnel: "Pattern2 Farbe" -> [_ w376]
      tunnel: w169 -> [w374 w375]
      frame False {
      }
      frame True {
        n164 = call "IMAQ Overlay Oval"("Color"=w376, "Bounding Rectangle"=w378, "Image"=w375) -> ("Image Out"=w377:T2)  [unwired: 7 in, 1 out]
      }
    }
    n165 = case shown="True" w282 {
      tunnel: w306 -> [_ w424]
      tunnel: [w420 w423] -> w271
      tunnel: "Pattern2 Farbe" -> [_ w422]
      tunnel: w172 -> [w420 w421]
      frame False {
      }
      frame True {
        n166 = call "IMAQ Overlay Oval"("Color"=w422, "Bounding Rectangle"=w424, "Image"=w421) -> ("Image Out"=w423:T2)  [unwired: 7 in, 1 out]
      }
    }
    n167 = call "Punkte_mit_linie_verbinden.vi"("Color"="Pattern1 Farbe", "Array"=w286, "dimension size"=w328, "Refnum in"=w271) -> ("Refnum out"=w295:T2)  [unwired: 7 in]
    n168 = call "linie_mit_pfeil.vi"("Richtungspfeillänge"="Länge des Pfeils", "Angle"=w285, "Color"="Pattern1 Farbe", "Boolean"=w283, "x"=w293, "y"=w292, "Refnum in"=w295) -> ("Refnum out"=w294:T2)  [unwired: 4 in]
    n169 = call "IMAQ Merge Overlay"("Image Src"=w294) -> ("Image Dst Out"=w312:T2)  [unwired: 9 in, 1 out]
    "Image 2" <- w312
    n170 = case shown="True" w302 {
      tunnel: w312 -> [_ w419]
      tunnel: w311 -> [w416 w418]
      tunnel: [w416 w417] -> w310
      frame False {
      }
      frame True {
        n171 = call "IMAQ AVI Write Frame"("Image"=w419, "Avi Refnum"=w418) -> ("Avi Refnum (duplicate)"=w417:T7)  [unwired: 8 in, 1 out]
      }
    }
  }
  n172 = Close File(refnum=w30) -> ()  [unwired: 1 in, 2 out]
  n173 = case shown="True" w84 {
    tunnel: w86 -> [_ w430]
    frame False {
    }
    frame True {
      n174 = call "IMAQ AVI Close"("Avi Refnum"=w430) -> ()  [unwired: 10 in, 1 out]
    }
  }
  n175 = call <vilib>:"IMAQdx Close Camera.vi"("Session In"=w108) -> ("error out"=w109:errorcluster)  [unwired: 10 in]
  n176 = call "IMAQ Dispose"("Image"=w105) -> ()  [unwired: 5 in, 1 out]
  n177 = call <vilib>:"Simple Error Handler.vi"("error in (no error)"=w109) -> ()  [unwired: 4 in, 5 out]
